vi "ge_String2Val.vi"(0 "String":string, 1 "ColType":T1, 2 "DefVal":u16=65535) -> (5 "Value":u16, 6 "Bridge Config (Conv)":u16(ring)=3 items=["Qtr Bridge I", "Qtr Bridge II", "Half Bridge I", "Half Bridge II", "Full Bridge I", "Full Bridge II", "Full Bridge III"])   [LabVIEW 2012]
uses:
  Custom Ctls Table/ge_ColType.ctl
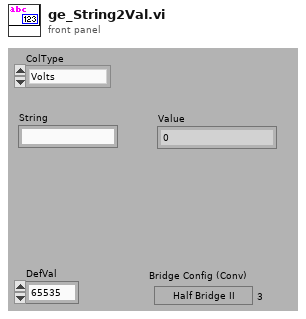
[diagram p1: front panel]
types:
  T1 = typedef "ge_ColType.ctl" = enum16{"Volts", "Amps", "Ohms", "TermCfg", "WireCfg", "Coup", "Slope", "Iex", "CalUnits", "ThrmUnits", "ThrmType", "CJCSrc", "BrdgType", "Strn Mode", "RTDType"}
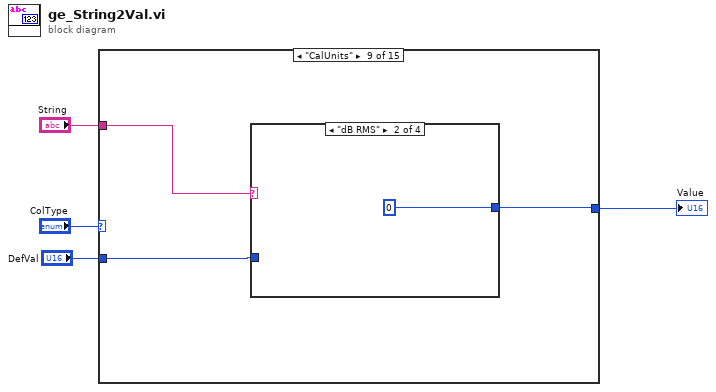
[diagram p0: block diagram]
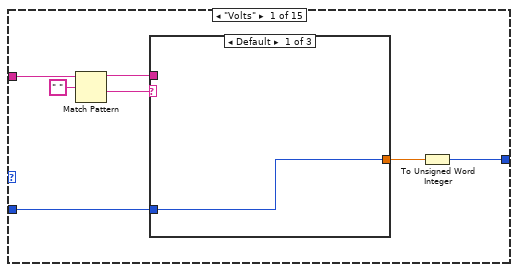
[diagram p2: hidden frame]
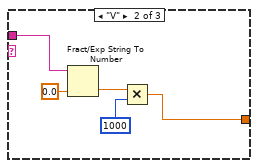
[diagram p3: hidden frame]
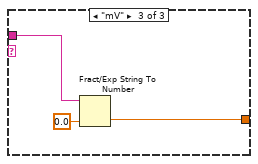
[diagram p4: hidden frame]
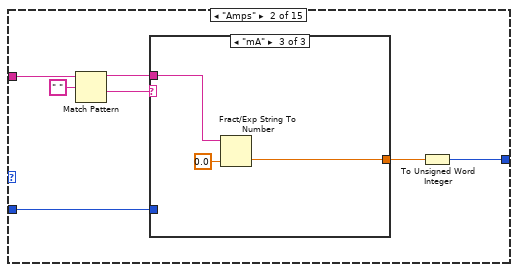
[diagram p5: hidden frame]
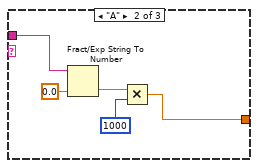
[diagram p7: hidden frame]
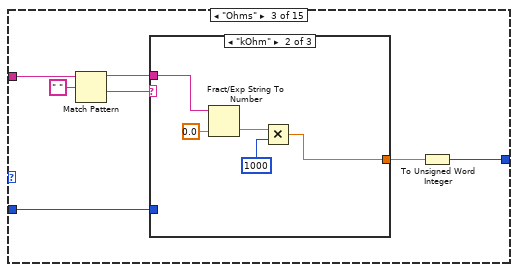
[diagram p8: hidden frame]
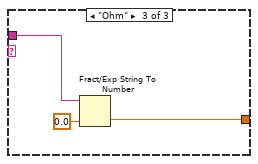
[diagram p10: hidden frame]
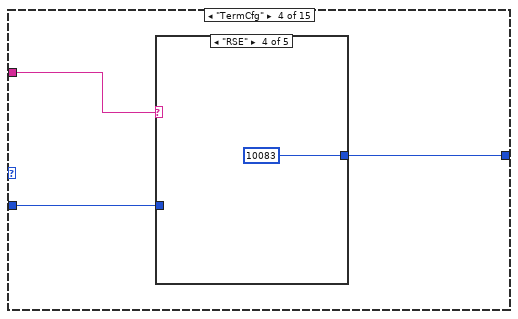
[diagram p11: hidden frame]
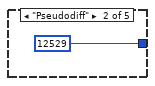
[diagram p13: hidden frame]
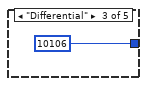
[diagram p14: hidden frame]
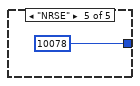
[diagram p15: hidden frame]
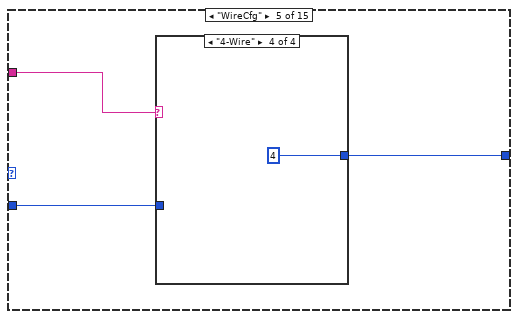
[diagram p16: hidden frame]
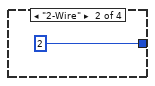
[diagram p18: hidden frame]
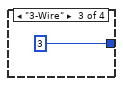
[diagram p19: hidden frame]
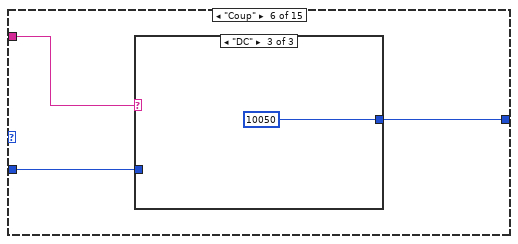
[diagram p20: hidden frame]
diagram:
  n1 = case shown="\"CalUnits\"" "ColType" {
    tunnel: "String" -> [w11 w27 w43 w55 w63 w70 w75 w83 w86 w94 w102 w114 w121 w140 w146]
    tunnel: "DefVal" -> [w7 w23 w39 w53 w61 w68 w76 _ w87 w93 w101 w113 w120 w139 w145]
    tunnel: [w5 w21 w37 w54 w62 w69 w74 w80 w85 w92 w100 w112 w119 w138 w144] -> w1
    frame "Volts" {
      n2 = Match Pattern(string=w11, regular expression=" ") -> (before substring=w8:string, after substring=w9:string)  [unwired: 1 in, 2 out]
      n3 = case shown="Default" w9 {
        tunnel: w8 -> [_ w16 w20]
        tunnel: [w12 w13 w19] -> w6
        tunnel: w7 -> [w12 _ _]
        frame Default {
        }
        frame "V" {
          n4 = Fract/Exp String To Number(string=w16, default (0 dbl)=0.0 ("default (0 I32)")) -> (number=w15:dbl)  [unwired: 2 in, 1 out]
          n5 = Multiply(x=w15, y=u16 1000) -> (x*y=w13:dbl)
        }
        frame "mV" {
          n6 = Fract/Exp String To Number(string=w20, default (0 dbl)=0.0 ("default (0 I32)")) -> (number=w19:dbl)  [unwired: 2 in, 1 out]
        }
      }
      n7 = To Unsigned Word Integer(number=w6) -> (unsigned 16bit integer=w5:u16)
    }
    frame "Amps" {
      n8 = Match Pattern(string=w27, regular expression=" ") -> (before substring=w24:string, after substring=w25:string)  [unwired: 1 in, 2 out]
      n9 = case shown="\"mA\"" w25 {
        tunnel: w24 -> [_ w32 w36]
        tunnel: [w28 w29 w35] -> w22
        tunnel: w23 -> [w28 _ _]
        frame Default {
        }
        frame "A" {
          n10 = Fract/Exp String To Number(string=w32, default (0 dbl)=0.0 ("default (0 I32)")) -> (number=w31:dbl)  [unwired: 2 in, 1 out]
          n11 = Multiply(x=w31, y=u16 1000) -> (x*y=w29:dbl)
        }
        frame "mA" {
          n12 = Fract/Exp String To Number(string=w36, default (0 dbl)=0.0 ("default (0 I32)")) -> (number=w35:dbl)  [unwired: 2 in, 1 out]
        }
      }
      n13 = To Unsigned Word Integer(number=w22) -> (unsigned 16bit integer=w21:u16)
    }
    frame "Ohms" {
      n14 = Match Pattern(string=w43, regular expression=" ") -> (before substring=w40:string, after substring=w41:string)  [unwired: 1 in, 2 out]
      n15 = case shown="\"kOhm\"" w41 {
        tunnel: w40 -> [_ w48 w52]
        tunnel: [w44 w45 w51] -> w38
        tunnel: w39 -> [w44 _ _]
        frame Default {
        }
        frame "kOhm" {
          n16 = Fract/Exp String To Number(string=w48, default (0 dbl)=0.0 ("default (0 I32)")) -> (number=w47:dbl)  [unwired: 2 in, 1 out]
          n17 = Multiply(x=w47, y=u16 1000) -> (x*y=w45:dbl)
        }
        frame "Ohm" {
          n18 = Fract/Exp String To Number(string=w52, default (0 dbl)=0.0 ("default (0 I32)")) -> (number=w51:dbl)  [unwired: 2 in, 1 out]
        }
      }
      n19 = To Unsigned Word Integer(number=w38) -> (unsigned 16bit integer=w37:u16)
    }
    frame "TermCfg" {
      n20 = case shown="\"RSE\"" w55 {
        tunnel: [w56 u16 12529 u16 10106 u16 10083 u16 10078] -> w54
        tunnel: w53 -> [w56 _ _ _ _]
        frame Default {
        }
        frame "Pseudodiff" {
        }
        frame "Differential" {
        }
        frame "RSE" {
        }
        frame "NRSE" {
        }
      }
    }
    frame "WireCfg" {
      n21 = case shown="\"4-Wire\"" w63 {
        tunnel: [w64 u16 2 u16 3 u16 4] -> w62
        tunnel: w61 -> [w64 _ _ _]
        frame Default {
        }
        frame "2-Wire" {
        }
        frame "3-Wire" {
        }
        frame "4-Wire" {
        }
      }
    }
    frame "Coup" {
      n22 = case shown="\"DC\"" w70 {
        tunnel: [w71 u16 10045 ("DefVal") u16 10050 ("DefVal")] -> w69
        tunnel: w68 -> [w71 _ _]
        frame Default {
        }
        frame "AC" {
        }
        frame "DC" {
        }
      }
    }
    frame "Slope" {
      n23 = case shown="\"Falling\"" w75 {
        tunnel: [w77 u16 0 ("DefVal") u16 1 ("DefVal")] -> w74
        tunnel: w76 -> [w77 _ _]
        frame Default {
        }
        frame "Rising" {
        }
        frame "Falling" {
        }
      }
    }
    frame "Iex" {
      n24 = Match Pattern(string=w83, regular expression=" ") -> (before substring=w81:string)  [unwired: 1 in, 3 out]
      n25 = Decimal String To Number(string=w81, default (0L)=u16 0 ("default (0 I32)")) -> (number=w80:u16)  [unwired: 1 in, 1 out]
    }
    frame "CalUnits" {
      n26 = case shown="\"dB RMS\"" w86 {
        tunnel: [w88 u16 0 ("DefVal") u16 1 ("DefVal") u16 2 ("DefVal")] -> w85
        tunnel: w87 -> [w88 _ _ _]
        frame Default {
        }
        frame "dB RMS" {
        }
        frame "EU Pk" {
        }
        frame "EU RMS" {
        }
      }
    }
    frame "ThrmUnits" {
      n27 = case shown="\"Deg R\"" w94 {
        tunnel: [w95 u16 10143 u16 10144 u16 10325 u16 10145] -> w92
        tunnel: w93 -> [w95 _ _ _ _]
        frame Default {
        }
        frame "Deg C" {
        }
        frame "Deg F" {
        }
        frame "Kelvins" {
        }
        frame "Deg R" {
        }
      }
    }
    frame "ThrmType" {
      n28 = case shown="\"J\"" w102 {
        tunnel: [w103 u16 10072 u16 10073 u16 10077 u16 10082 u16 10085 u16 10086 u16 10047 u16 10055] -> w100
        tunnel: w101 -> [w103 _ _ _ _ _ _ _ _]
        frame Default {
        }
        frame "J" {
        }
        frame "K" {
        }
        frame "N" {
        }
        frame "R" {
        }
        frame "S" {
        }
        frame "T" {
        }
        frame "B" {
        }
        frame "E" {
        }
      }
    }
    frame "CJCSrc" {
      n29 = case shown="\"Built-In\"" w114 {
        tunnel: [w115 u16 10116 u16 10200] -> w112
        tunnel: w113 -> [w115 _ _]
        frame Default {
        }
        frame "Const Val" {
        }
        frame "Built-In" {
        }
      }
    }
    frame "BrdgType" {
      n30 = case shown="\"Half Bridge II\"" w121 {
        tunnel: [w123 u16 10183 u16 10184 u16 10185 u16 10188 u16 10189 u16 10271 u16 10272] -> w119
        tunnel: w120 -> [w123 _ _ _ _ _ _ _]
        tunnel: [u16 0 ("Bridge Configuration\n(3:Half Bridge II)") w124 w126 w128 w130 w132 w134 w136] -> w118
        frame Default {
        }
        frame "Full Bridge I" {
          w124 = u16 4 items=["Qtr Bridge I", "Qtr Bridge II", "Half Bridge I", "Half Bridge II", "Full Bridge I", "Full Bridge II", "Full Bridge III"] ("Bridge Configuration\n(3:Half Bridge II)")
        }
        frame "Full Bridge II" {
          w126 = u16 5 items=["Qtr Bridge I", "Qtr Bridge II", "Half Bridge I", "Half Bridge II", "Full Bridge I", "Full Bridge II", "Full Bridge III"] ("Bridge Configuration\n(3:Half Bridge II)")
        }
        frame "Full Bridge III" {
          w128 = u16 6 items=["Qtr Bridge I", "Qtr Bridge II", "Half Bridge I", "Half Bridge II", "Full Bridge I", "Full Bridge II", "Full Bridge III"] ("Bridge Configuration\n(3:Half Bridge II)")
        }
        frame "Half Bridge I" {
          w130 = u16 2 items=["Qtr Bridge I", "Qtr Bridge II", "Half Bridge I", "Half Bridge II", "Full Bridge I", "Full Bridge II", "Full Bridge III"] ("Bridge Configuration\n(3:Half Bridge II)")
        }
        frame "Half Bridge II" {
          w132 = u16 3 items=["Qtr Bridge I", "Qtr Bridge II", "Half Bridge I", "Half Bridge II", "Full Bridge I", "Full Bridge II", "Full Bridge III"] ("Bridge Configuration\n(3:Half Bridge II)")
        }
        frame "Quarter Bridge I" {
          w134 = u16 0 items=["Qtr Bridge I", "Qtr Bridge II", "Half Bridge I", "Half Bridge II", "Full Bridge I", "Full Bridge II", "Full Bridge III"] ("Bridge Configuration\n(3:Half Bridge II)")
        }
        frame "Quarter Bridge II" {
          w136 = u16 1 items=["Qtr Bridge I", "Qtr Bridge II", "Half Bridge I", "Half Bridge II", "Full Bridge I", "Full Bridge II", "Full Bridge III"] ("Bridge Configuration\n(3:Half Bridge II)")
        }
      }
      "Bridge Config (Conv)" <- w118
    }
    frame "Strn Mode" {
      n31 = case shown="\"High Range\"" w140 {
        tunnel: [w141 u16 0 u16 1] -> w138
        tunnel: w139 -> [w141 _ _]
        frame Default {
        }
        frame "High Res" {
        }
        frame "High Range" {
        }
      }
    }
    frame "RTDType" {
      n32 = case shown="Default" w146 {
        tunnel: [w147 u16 12481 u16 10071 u16 12482 u16 10069 u16 10053 u16 12483] -> w144
        tunnel: w145 -> [w147 _ _ _ _ _ _]
        frame Default {
        }
        frame "Pt3750" {
        }
        frame "Pt3851" {
        }
        frame "Pt3911" {
        }
        frame "Pt3916" {
        }
        frame "Pt3920" {
        }
        frame "Pt3928" {
        }
      }
    }
  }
  "Value" <- w1
